vi "Configure ARB CDWell Stop.vi"(8 "error in":errorcluster, 11 "VISA resource name":refnum<visa-resource-name>) -> (0 "error out":errorcluster, 3 "VISA resource name out":refnum<visa-resource-name>)   [LabVIEW 2024, in "IT-M3900C.lvlib"]
doc: "This command sets the abort waveform (abort after all the data has been executed, as opposed to abort, which is to stop immediately)."
uses:
  IT-M3900C.lvlib
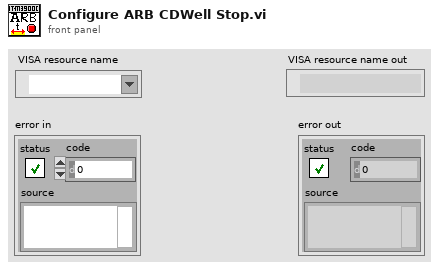
[diagram p1: front panel]
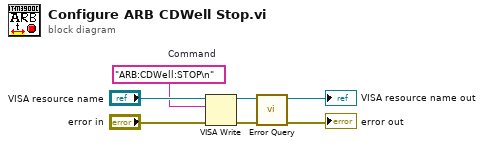
[diagram p0: block diagram]
diagram:
  w5 = "ARB:CDWell:STOP\n"  # Command
  n1 = VISA Write(VISA resource name="VISA resource name", write buffer=w5, error in (no error)="error in") -> (VISA resource name out=w3:refnum<visa-resource-name>, error out=w4:errorcluster)  [unwired: 1 out]
  n2 = call "Error Query.vi"("error in"=w4, "VISA resource name"=w3) -> ("error out"=→"error out":errorcluster, "VISA resource name out"=→"VISA resource name out":refnum<visa-resource-name>)  [unwired: 6 in, 2 out]
